vi "AnotherTestingGUI.vi"() -> ()   [LabVIEW 2018]
uses:
  Type_Def/Type_Def ControlState.ctl
panel:
  in  "ServivcePush":bool
  in  "Force Idle":bool
  in  "stop":bool
  in  "Vent":bool
  in  "Service":bool
  in  "Ready":bool
  in  "SystemCheck":bool
  in  "Shutdown":bool
  out "CurrentState":T1
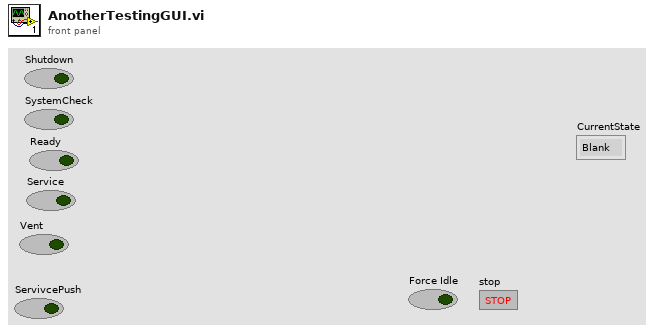
[diagram p1: front panel]
types:
  T1 = typedef "Type_Def ControlState.ctl" = enum16{"Blank", "Systems Check", "Idle", "Ready", "Pushing", "CrawlingPrecharge", "Braking", "Fault", "Boot Up", "Unpowered", "Crawling", "Shutdown", "Service Push", "Service Wait", "Vent", "Precharge", "Cooldown"}
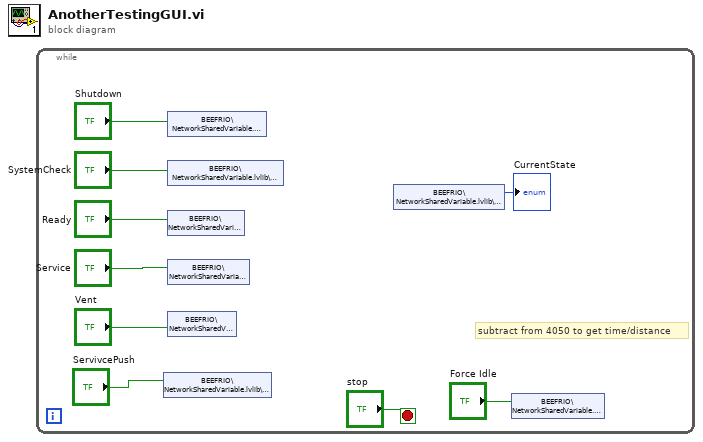
[diagram p0: block diagram]
diagram:
  n1 = while {
    stop <- "stop" stop-if-true
    # "subtract from 4050 to get time/distance"
    n2 = shared-variable "BEEFRIO\\NetworkSharedVariable.lvlib\\ServicePush"("ServivcePush") -> ()  [unwired: 1 in, 1 out]
    n3 = shared-variable "BEEFRIO\\NetworkSharedVariable.lvlib\\Shutdown"("Shutdown") -> ()  [unwired: 1 in, 1 out]
    n4 = shared-variable "BEEFRIO\\NetworkSharedVariable.lvlib\\SystemCheck"("SystemCheck") -> ()  [unwired: 1 in, 1 out]
    n5 = shared-variable "BEEFRIO\\NetworkSharedVariable.lvlib\\Ready"("Ready") -> ()  [unwired: 1 in, 1 out]
    n6 = shared-variable "BEEFRIO\\NetworkSharedVariable.lvlib\\Service"("Service") -> ()  [unwired: 1 in, 1 out]
    n7 = shared-variable "BEEFRIO\\NetworkSharedVariable.lvlib\\Vent"("Vent") -> ()  [unwired: 1 in, 1 out]
    n8 = shared-variable "BEEFRIO\\NetworkSharedVariable.lvlib\\CurrentState"() -> (→"CurrentState":T1)  [unwired: 1 in, 1 out]
    n9 = shared-variable "BEEFRIO\\NetworkSharedVariable.lvlib\\ForceIdle"("Force Idle") -> ()  [unwired: 1 in, 1 out]
  }
